vi "WriteDBfile.vi"(3 "String IN":string, 5 "UploadRawData?":bool) -> (6 "error out":errorcluster, 7 "RawDataFileName":string, 8 "DBFileName OUT":string)   [LabVIEW 2013]
uses:
  global/newtest.vi
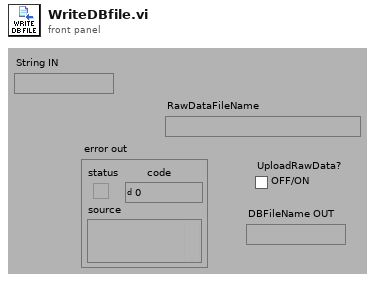
[diagram p1: front panel]
types:
  T1 = enum16{"open", "open or create", "create or replace", "create"}
  T2 = cluster{"Serial Number":string, "Operator":string, "Run number":string, "Date":string, "lookup":u16, "Device type":string}
  T3 = cluster{"Manufacturers":string[], "Users":string[], "Device Categories":string[], "MeasurementTypeDirs":string[], "PCNames":string[], "FilePaths":string[], "ThisPCNumber":string, "Full PC Names":string[], "SCTDB Files":string[], "Backuplog directory":string, "Lookup tables":string[], "Projects":string[], "ThisProjectNumber":string, "Institute":string, "java classpath":string, "WWW directories":string[], "BatchFiles":string[], "Logfiles":string[]}
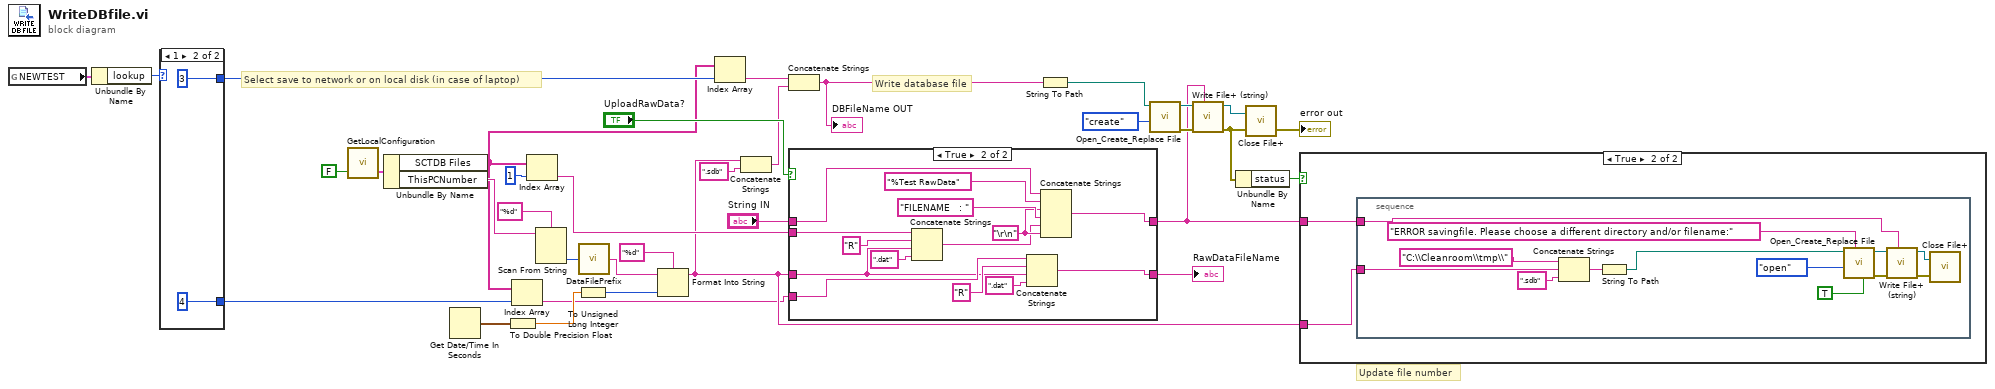
[diagram p0: block diagram]
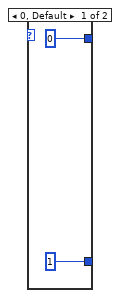
[diagram p2: hidden frame]
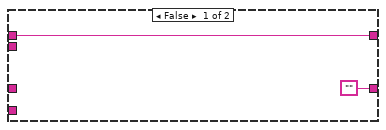
[diagram p4: hidden frame]
diagram:
  # "Select save to network or on local disk (in case of laptop)"
  # "Update file number"
  # "Write database file"
  n1 = global read "newtest.vi" "NEWTEST"() -> (w11:T2)
  n2 = Unbundle By Name(w11) -> ("lookup"=w10:u16)
  n3 = case shown="1" w10 {
    tunnel: [0 3] -> w35
    tunnel: [1 4] -> w7
    frame 0, Default {
    }
    frame 1 {
    }
  }
  n4 = call "GetLocalConfiguration.vi"("force read?"=FALSE) -> ("Local Configuration"=w24:T3)  [unwired: 2 in]
  n5 = Unbundle By Name(w24) -> ("SCTDB Files"=w6:string[], "ThisPCNumber"=w21:string)
  n6 = Get Date/Time In Seconds() -> (seconds since 1Jan1904=w2:timestamp)
  n7 = To Double Precision Float(number=w2) -> (double precision float=w19:dbl)
  n8 = Index Array(array=w6, index=w7) -> (element=w8:string)
  n9 = Index Array(array=w6, index=1) -> (element=w26:string)
  n10 = Scan From String(format string="%d", input string=w21) -> (output 1=w22:i32)  [unwired: 3 in, 3 out]
  n11 = To Unsigned Long Integer(number=w19) -> (unsigned 32bit integer=w18:u32)
  n12 = call "DataFilePrefix.vi"("PC number IN"=w22) -> ("File prefix OUT"=w20:string)
  n13 = Format Into String(format string="%d", initial string=w20, w18) -> (resulting string=w12:string)  [unwired: 1 in, 1 out]
  n14 = Index Array(array=w6, index=w35) -> (element=w5:string)
  n15 = Concatenate Strings(w12, ".sdb") -> (w4:string)
  n16 = Concatenate Strings(w5, w4) -> (w3:string)
  "DBFileName OUT" <- w3
  n17 = case shown="True" "UploadRawData?" {
    tunnel: "String IN" -> [w41 w51]
    tunnel: [w41 w52] -> w13
    tunnel: w12 -> [_ w44]
    tunnel: w26 -> [_ w53]
    tunnel: ["" w42] -> w25
    tunnel: w8 -> [_ w45]
    frame False {
    }
    frame True {
      w49 = "\r\n"
      n18 = Concatenate Strings(w53, "R", w44, ".dat") -> (w43:string)
      n19 = Concatenate Strings(w45, "R", w44, ".dat") -> (w42:string)
      n20 = Concatenate Strings(w51, "%Test RawData", w49, "FILENAME   : ", w43, w49) -> (w52:string)
    }
  }
  "RawDataFileName" <- w25
  n21 = String To Path(string=w3) -> (path=w33:path)
  n22 = call <vilib>:"Open_Create_Replace File.vi"("function (open:0)"=T1."create", "file path"=w33) -> ("error out"=w29:errorcluster, "refnum"=w31:refnum<file>)  [unwired: 6 in, 2 out]
  n23 = call <vilib>:"Write File+ (string).vi"("string"=w13, "error in (no error)"=w29, "refnum"=w31) -> ("error out"=w15:errorcluster, "dup refnum"=w30:refnum<file>)  [unwired: 4 in, 1 out]
  n24 = Unbundle By Name(w15) -> ("status"=w14:bool)
  n25 = call <vilib>:"Close File+.vi"("error in (no error)"=w15, "refnum"=w30) -> ("error out"=→"error out":errorcluster)  [unwired: 3 in, 2 out]
  n26 = case shown="True" w14 {
    tunnel: w13 -> [_ w57]
    tunnel: w12 -> [_ w56]
    frame False {
    }
    frame True {
      n27 = stacked-sequence {
        tunnel: w57 -> [w66]
        tunnel: w56 -> [w63]
        frame #0 {
          n28 = Concatenate Strings("C:\\Cleanroom\\tmp\\", w63, ".sdb") -> (w60:string)
          n29 = String To Path(string=w60) -> (path=w61:path)
          n30 = call <vilib>:"Open_Create_Replace File.vi"("advisory dialog? (display:T)"=TRUE, "prompt"="ERROR savingfile. Please choose a different directory and/or filename:", "function (open:0)"=T1."open", "file path"=w61) -> ("error out"=w65:errorcluster, "refnum"=w68:refnum<file>)  [unwired: 4 in, 2 out]
          n31 = call <vilib>:"Write File+ (string).vi"("string"=w66, "error in (no error)"=w65, "refnum"=w68) -> ("error out"=w64:errorcluster, "dup refnum"=w67:refnum<file>)  [unwired: 4 in, 1 out]
          n32 = call <vilib>:"Close File+.vi"("error in (no error)"=w64, "refnum"=w67) -> ()  [unwired: 3 in, 3 out]
        }
      }
    }
  }
